vi "DFD Remez Design.vi"(5 "minimum order":enum32{"User Defined", "MinEven", "MinOdd"}(ring), 6 "fs [Hz]":dbl=1.0 format="%.2f", 7 "filter type":T1, 8 "error in (no error)":errorcluster, 9 "freqs of exact gain [Hz]":dbl[](array[numeric]), 10 "band specs":T2[](array[typedef])=[{"band specification"=[{"freq"=0.0, "amplitude"=1.0, "weight"=1.0}, {"freq"=0.2, "amplitude"=1.0, "weight"=1.0}], "ripple constraint"=0.0}, {"band specification"=[{"freq"=0.3, "amplitude"=0.0, "weight"=1.0}, {"freq"=0.5, "amplitude"=0.0, "weight"=1.0}], "ripple constraint"=0.0}], 11 "order":i32=20) -> (0 "error out":errorcluster, 2 "actual ripples":dbl[](array[numeric]), 3 "filter out":T3={"mSRate_Fs"=1.0, "mSRate_Version"="2.0", "mSRate_Comments"="", "mSRate_OrgCoef"={"type"=enum."Undefined", "gain"=1.0, "coef a (k)"=[], "coef b (v)"=[]}, "mSRate_CurCoef"={"type"=enum."Undefined", "gain"=1.0, "coef a (k)"=[], "coef b (v)"=[]}, "mSRate_Quantized?"=FALSE, "mSRate_QCoef"={"type"=enum."Undefined", "gain"=1.0, "coef a (k)"=[], "coef b (v)"=[]}, "mSRate_QSettings"=[], "mSRate_Order"=0, "mSRate_Scaling"={"mSRate_ScaleByPowerOf2?"=FALSE, "mSRate_ScaleType"=enum."No Norm"}} {"mSRate_QSettings"."source" items=["Coef a/k"=0, "Coef b/v"=7, "Input"=1, "Output"=2, "Multiplicand"=3, "Product"=4, "Sum"=5, "Delay"=6, "Gain"=8]})   [LabVIEW 2017, in "NI_DigFilterLicensed.lvlib"]
doc: "Creates an equi-ripple filter using the Remez exchange method."
uses:
  <vilib>/addons/Digital Filter Design/NI_DigFilterLicensed.lvlib
  <vilib>/addons/Digital Filter Design/_Objects.llb/DFD Filter Obj.ctl
  <vilib>/addons/Digital Filter Design/_Objects.llb/DFD Filter Coef.ctl
  <vilib>/addons/Digital Filter Design/_Objects.llb/DFD Filter Structure Type Selector.ctl
  <vilib>/addons/Digital Filter Design/_Objects.llb/dfd_Internal Quantization Settings.ctl
  <vilib>/addons/Digital Filter Design/_Objects.llb/dfd_Internal Quantization Srcs.ctl
  <vilib>/addons/Digital Filter Design/_Objects.llb/DFD Coef Norm Type.ctl
  <vilib>/addons/Digital Filter Design/_Objects.llb/DFD Adv Band Spec.ctl
  <vilib>/addons/Digital Filter Design/_REMEZ.llb/remez_fir filter type.ctl
  <vilib>/addons/Digital Filter Design/NI_DigFilter_Design.lvlib
panel:
  # "freq"
  # "amplitude"
  # "weight"
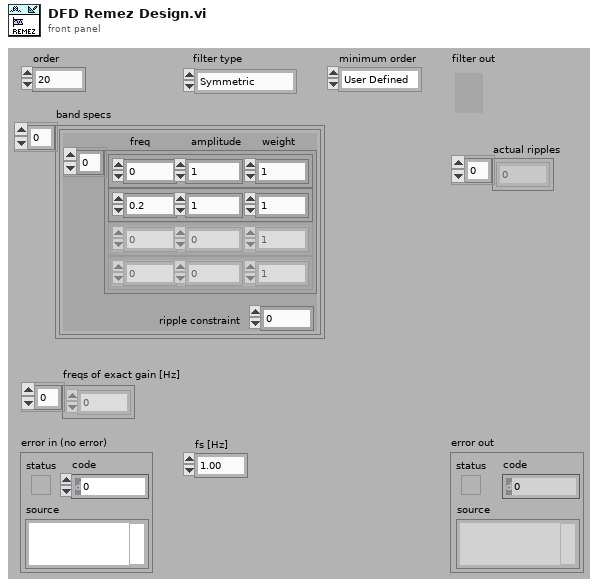
[diagram p1: front panel]
types:
  T1 = typedef "NI_DigFilterLicensed.lvlib/remez_fir filter type.ctl" = enum32{"Symmetric", "Antisymmetric", "Differentiator", "Hilbert", "Minimum Phase", "Maximum Phase"}
  T2 = typedef "NI_DigFilterLicensed.lvlib/DFD Adv Band Spec.ctl" = cluster{"band specification":cluster{"freq":dbl, "amplitude":dbl, "weight":dbl}[], "ripple constraint":dbl}
  T3 = typedef "NI_DigFilterLicensed.lvlib/DFD Filter Obj.ctl" = cluster{"mSRate_Fs":dbl, "mSRate_Version":string, "mSRate_Comments":string, "mSRate_OrgCoef":T4, "mSRate_CurCoef":T4, "mSRate_Quantized?":bool, "mSRate_QCoef":T4, "mSRate_QSettings":T6[], "mSRate_Order":i32, "mSRate_Scaling":cluster{"mSRate_ScaleByPowerOf2?":bool, "mSRate_ScaleType":T8}}
  T4 = typedef "NI_DigFilterLicensed.lvlib/DFD Filter Coef.ctl" = cluster{"type":T5, "gain":dbl, "coef a (k)":dbl[], "coef b (v)":dbl[]}
  T5 = typedef "NI_DigFilterLicensed.lvlib/DFD Filter Structure Type Selector.ctl" = enum16{"Undefined", "FIR Direct Form", "FIR Direct Form Transposed", "FIR Symmetric", "FIR Antisymmetric", "IIR Direct Form I", "IIR Direct Form I Transposed", "IIR Direct Form II", "IIR Direct Form II Transposed", "IIR Cascaded Second Order Sections Form I", "IIR Cascaded Second Order Sections Form I Transposed", "IIR Cascaded Second Order Sections Form II", "IIR Cascaded Second Order Sections Form II Transposed", "Lattice Allpass (basic sections)", "Lattice Allpass (one multiplier sections)", "Lattice Allpass (normalized sections)", "Lattice AR (basic sections)", "Lattice AR (one multiplier sections)", "Lattice AR (normalized sections)", "Lattice MA (minimum phase)", "Lattice MA (maximum phase)", "Lattice ARMA (basic sections)", "Lattice ARMA (one multiplier sections)", "Lattice ARMA (normalized sections)"}
  T6 = typedef "NI_DigFilterLicensed.lvlib/dfd_Internal Quantization Settings.ctl" = cluster{"source":T7, "wl":i16, "iwl":i16, "overflow mode":enum16{"Saturation", "Wrap"}, "rounding mode":enum16{"Nearest", "Truncation"}, "signed?":bool}
  T7 = typedef "NI_DigFilterLicensed.lvlib/dfd_Internal Quantization Srcs.ctl" = u16
  T8 = typedef "NI_DigFilterLicensed.lvlib/DFD Coef Norm Type.ctl" = enum16{"No Norm", "Time Domain 1-Norm", "Time Domain 2-Norm", "Time Domain Inf-Norm"}
  T9 = typedef "remez_band specification.ctl" = T10[]
  T10 = typedef "remez_single band description.ctl" = cluster{"points":cluster{"f":dbl, "A":dbl, "W":dbl, "forced gain?":bool}[], "band weight":dbl, "constraint":dbl, "ripple idx":i32, "in band weight option":enum16{"ignore", "linear interpolation", "const amplitude %"}}
  T11 = typedef "remez_fir order and types.ctl" = cluster{"# of taps":i32, "filter type":T1, "minimum order":enum32{"user defined", "minEven", "minOdd"}}
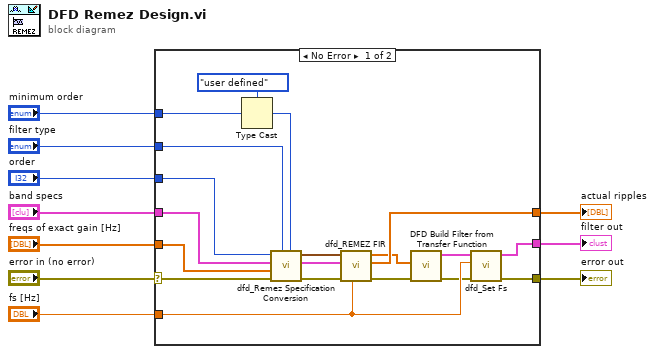
[diagram p0: block diagram]
diagram:
  n1 = case shown="No Error" "error in (no error)" {
    selector: "error in (no error)" -> [w11 w30]
    tunnel: [w29 _] -> w10
    tunnel: "fs [Hz]" -> [w28 _]
    tunnel: [w27 _] -> w8
    tunnel: "freqs of exact gain [Hz]" -> [w23 _]
    tunnel: "band specs" -> [w21 _]
    tunnel: "order" -> [w20 _]
    tunnel: "filter type" -> [w19 _]
    tunnel: "minimum order" -> [w18 _]
    tunnel: [w15 w30] -> w2
    frame No Error {
      n2 = Type Cast(type=enum32{"user defined", "minEven", "minOdd"}."user defined" ("minimum order"), x=w18) -> (*(type *) &x=w13:enum32{"user defined", "minEven", "minOdd"})
      n3 = call <vilib>:"dfd_Remez Specification Conversion.vi"("minimum order"=w13, "phase option"=w19, "error in (no error)"=w11, "freq of forced gain [Hz]"=w23, "band parameters"=w21, "order"=w20) -> ("error out"=w22:errorcluster, "band specification"=w16:T9, "order and type"=w17:T11)  [unwired: 3 out]
      n4 = call <vilib>:"dfd_REMEZ FIR.vi"("fs"=w28, "error in (no error)"=w22, "band specification"=w16, "order and type"=w17) -> ("error out"=w26:errorcluster, "actual ripples"=w27:dbl[], "h"=w14:dbl[])  [unwired: 3 in, 2 out]
      n5 = call <vilib>:"DFD Build Filter from Transfer Function.vi"("error in (no error)"=w26, "numerator"=w14) -> ("error out"=w24:errorcluster, "filter out"=w25:T3)  [unwired: 2 in, 6 out]
      n6 = call <vilib>:"dfd_Set Fs.vi"("error in (no error)"=w24, "fs [Hz]"=w28, "filter in"=w25) -> ("error out"=w15:errorcluster, "filter out"=w29:T3)  [unwired: 7 out]
    }
    frame Error {
    }
  }
  "filter out" <- w10
  "error out" <- w2
  "actual ripples" <- w8
